vi "get UI reference.vi"(8 "error in":errorcluster, 11 "protection settings in":refnum<class "protection settings.lvclass">) -> (0 "error out":errorcluster, 2 "VI Refnum":refnum<vi>, 3 "protection settings out":refnum<class "protection settings.lvclass">)   [LabVIEW 2013, in "protection settings.lvclass"]
uses:
  protection settings.lvclass
  VI modification.lvclass
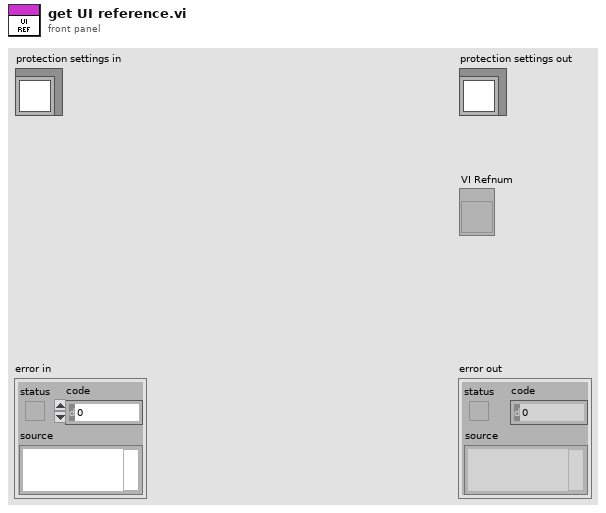
[diagram p1: front panel]
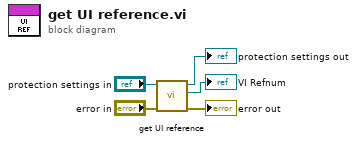
[diagram p0: block diagram]
diagram:
  n1 = call-parent "get UI reference.vi"("error in"="error in", "VI modification in"="protection settings in") -> ("error out"=→"error out":errorcluster, "VI Refnum"=→"VI Refnum":refnum<vi>, "VI modification out"=→"protection settings out":refnum<class "protection settings.lvclass">)  [unwired: 7 in]
